vi "Graph Range Update.vi"(4 "Axis":enum16{"X-Scale", "Y-Scale", "Z-Scale"}(ring), 6 "NewRange":T1, 8 "error in (no error)":errorcluster, 11 "3D Plot.lvclass in":refnum<class "3D Plot.lvclass">) -> (0 "error out":errorcluster, 3 "3D Plot.lvclass out":refnum<class "3D Plot.lvclass">)   [LabVIEW 2017, in "3D Plot.lvclass"]
uses:
  <vilib>/Math Plots/3D Math Plots/3D Plot/3D Plot/3D Plot.lvclass
  <vilib>/Math Plots/3D Math Plots/3D Plot/3D Plot/3D Plot.lvclass/3D Plot.ctl
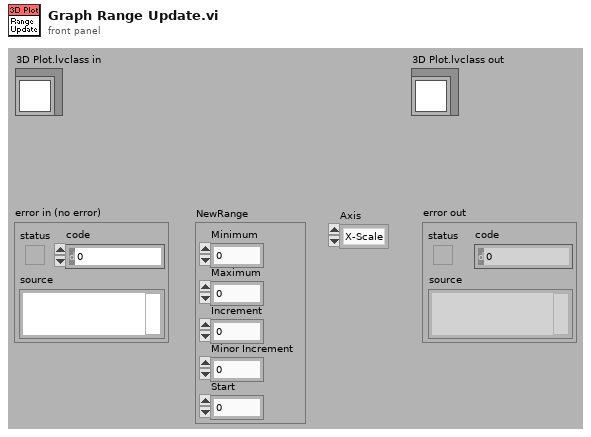
[diagram p1: front panel]
types:
  T1 = cluster{"Minimum":dbl, "Maximum":dbl, "Increment":dbl, "Minor Increment":dbl, "Start":dbl}
  T2 = enum32{"Towards X-Y Plane", "Towards X-Z Plane", "Towards Y-Z Plane", "User Defined"}
  T3 = typedef "3D Plot.lvclass/Range Property.ctl" = cluster{"Range Cluster":T4, "Auto Range":cluster{"Auto Range X":bool, "Auto Range Y":bool, "Auto Range Z":bool}, "Inverted":cluster{"Inverted X":bool, "Inverted Y":bool, "Inverted Z":bool}, "Logarithm":cluster{"Logarithm X":bool, "Logarithm Y":bool, "Logarithm Z":bool}}
  T4 = typedef "3D Plot.lvclass/Range Clusters.ctl" = cluster{"X Range":cluster{"Max X":sgl, "Min X":sgl}, "Y Range":cluster{"Max Y":sgl, "Min Y":sgl}, "Z Range":cluster{"Max Z":sgl, "Min Z":sgl}}
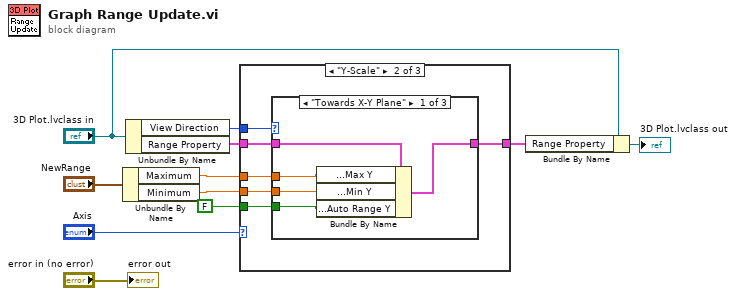
[diagram p0: block diagram]
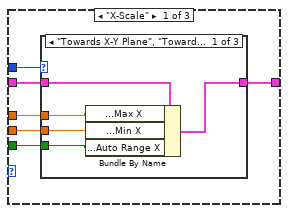
[diagram p2: hidden frame]
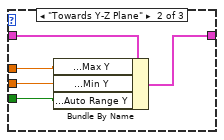
[diagram p3: hidden frame]
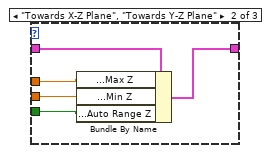
[diagram p5: hidden frame]
diagram:
  n1 = Unbundle By Name("NewRange") -> ("Maximum"=w8:dbl, "Minimum"=w7:dbl)
  n2 = Unbundle By Name("3D Plot.lvclass in") -> ("View Direction"=w10:T2, "Range Property"=w6:T3)
  n3 = case shown="\"Y-Scale\"" "Axis" {
    tunnel: [w17 w34 w46] -> w2
    tunnel: w10 -> [w16 w33 _]
    tunnel: w8 -> [w15 w32 _]
    tunnel: w7 -> [w14 w31 _]
    tunnel: w6 -> [w13 w30 w46]
    tunnel: FALSE -> [w12 w29 _]
    frame "X-Scale" {
      n4 = case shown="\"Towards X-Y Plane\", \"Towards X-Z Plane\"" w16 {
        tunnel: w15 -> [w21 w26 _]
        tunnel: w14 -> [w20 w25 _]
        tunnel: w13 -> [w22 w27 w28]
        tunnel: [w19 w24 w28] -> w17
        tunnel: w12 -> [w18 w23 _]
        frame "Towards X-Y Plane", "Towards X-Z Plane" {
          n5 = Bundle By Name(cluster=w22, "Range Cluster.X Range.Max X"=w21, "Range Cluster.X Range.Min X"=w20, "Auto Range.Auto Range X"=w18) -> (w19:T3)
        }
        frame "Towards Y-Z Plane" {
          n6 = Bundle By Name(cluster=w27, "Range Cluster.Y Range.Max Y"=w26, "Range Cluster.Y Range.Min Y"=w25, "Auto Range.Auto Range Y"=w23) -> (w24:T3)
        }
        frame "User Defined", Default {
        }
      }
    }
    frame "Y-Scale" {
      n7 = case shown="\"Towards X-Y Plane\"" w33 {
        tunnel: w32 -> [w38 w43 _]
        tunnel: w31 -> [w37 w42 _]
        tunnel: w30 -> [w39 w44 w45]
        tunnel: [w36 w41 w45] -> w34
        tunnel: w29 -> [w35 w40 _]
        frame "Towards X-Y Plane" {
          n8 = Bundle By Name(cluster=w39, "Range Cluster.Y Range.Max Y"=w38, "Range Cluster.Y Range.Min Y"=w37, "Auto Range.Auto Range Y"=w35) -> (w36:T3)
        }
        frame "Towards X-Z Plane", "Towards Y-Z Plane" {
          n9 = Bundle By Name(cluster=w44, "Range Cluster.Z Range.Max Z"=w43, "Range Cluster.Z Range.Min Z"=w42, "Auto Range.Auto Range Z"=w40) -> (w41:T3)
        }
        frame "User Defined", Default {
        }
      }
    }
    frame "Z-Scale", Default {
    }
  }
  n10 = Bundle By Name(cluster="3D Plot.lvclass in", "Range Property"=w2) -> (→"3D Plot.lvclass out":refnum<class "3D Plot.lvclass">)
  "error out" <- "error in (no error)"
